vi "S Gate.vi"(2 "v Ctrl in":refnum<class "CtrlLine.lvclass">, 7 "QuWire in":refnum<class "QuWire.lvclass">, 13 "^ Ctrl in":refnum<class "CtrlLine.lvclass">) -> (8 "QuWire out":refnum<class "QuWire.lvclass">)   [LabVIEW 2020]
doc: "S Gate\n\nApplies a pi/2 phase shift. \nIt is the square root of the Z gate (Z = S^2). Leaves |0> unchanged and maps |1> to i|1>.\n\nMatrix: [[ 1, 0], [ 0, i]]"
uses:
  QuSim/QuWire/QuWire.lvclass
  QuSim/QuWire/CtrlLine/CtrlLine.lvclass
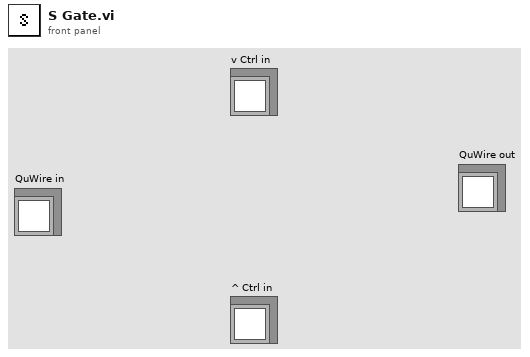
[diagram p1: front panel]
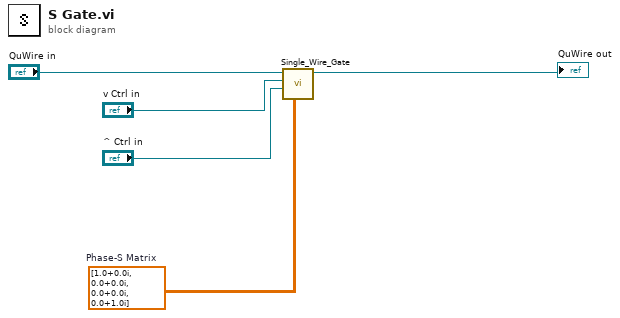
[diagram p0: block diagram]
diagram:
  w1 = cdb[][] [[1.0+0.0i, 0.0+0.0i], [0.0+0.0i, 0.0+1.0i]]  # Phase-S Matrix
  n1 = call "Single_Wire_Gate.vi"("2x2 Unitary Matrix"=w1, "d CtrlLine in"="^ Ctrl in", "u CtrlLine in"="v Ctrl in", "QuWire in"="QuWire in") -> ("QuWire out"=→"QuWire out":refnum<class "QuWire.lvclass">)  [unwired: 6 in, 1 out]
